vi "LVClass_WavefrontCorrector Get amplitude.vi"(0 "WavefrontCorrector in":refnum<class "WavefrontCorrector.lvclass">, 5 "Absolute Positions":T1, 11 "error in (no error)":errorcluster) -> (4 "WavefrontCorrector out":refnum<class "WavefrontCorrector.lvclass">, 6 "Absolute Positions OUT":T1, 8 "command_amplitude":sgl, 15 "error out":errorcluster)   [LabVIEW 2020, in "WavefrontCorrector.lvclass"]
doc: "Assert if requested absolute positions satisfy current preferences.\n\n--------------------------------------------------------------------------------\n\n<B>correctorIn </B> : WavefrontCorrector object.\n<B>correctorOut </B> : WavefrontCorrector object.\n<B>position </B> : Requested absolutes positions.\n<B>ErrorIn </B> : Error\n<B>ErrorOut </B> : Error\n\n--------------------------------------------------------------------------------"
uses:
  WavefrontCorrector.lvclass
  Wavefront Corrector Position.ctl
  WavefrontCorrector.lvclass/WavefrontCorrector.ctl
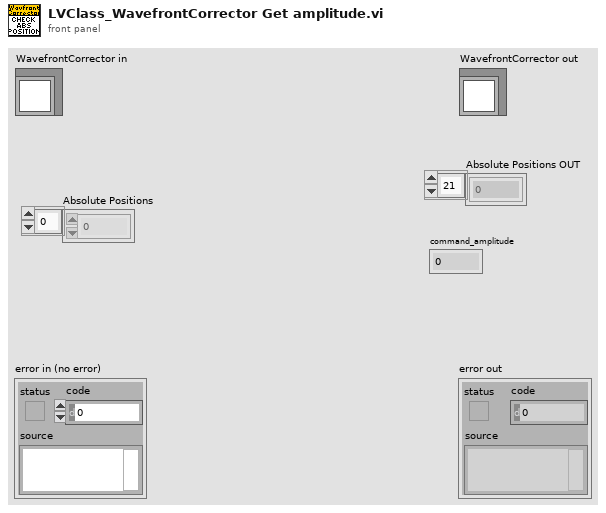
[diagram p1: front panel]
types:
  T1 = typedef "Wavefront Corrector Position.ctl" = sgl[]
  T2 = typedef "ClassID.ctl" = i64
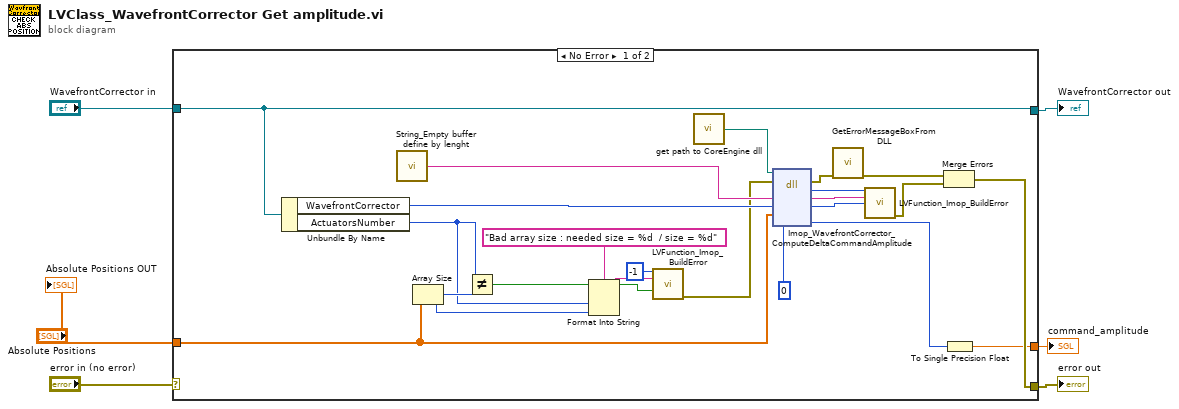
[diagram p0: block diagram]
diagram:
  n1 = case shown="No Error" "error in (no error)" {
    selector: "error in (no error)" -> [_ w30]
    tunnel: [w20 w30] -> w3
    tunnel: [w19 w29] -> w4
    tunnel: "WavefrontCorrector in" -> [w19 w29]
    tunnel: "Absolute Positions" -> [w11 _]
    tunnel: [w8 _] -> w1
    frame No Error {
      n2 = Unbundle By Name(w19) -> ("WavefrontCorrector"=w21:T2, "ActuatorsNumber"=w13:i32)
      n3 = call "String_Empty buffer define by lenght.vi"() -> ("Empty buffer"=w26:string)  [unwired: 1 in]
      n4 = Array Size(array=w11) -> (size(s)=w16:i32)
      n5 = Not Equal?(x=w13, y=w16) -> (x != y?=w15:bool)
      n6 = Format Into String(format string="Bad array size : needed size = %d  / size = %d" ("String to Prepend to source (\"\")"), w13, w16) -> (resulting string=w17:string)  [unwired: 2 in, 1 out]
      n7 = call "LVFunction_Imop_BuildError.vi"("code"=-1, "String to Prepend to source (\"\")"=w17, "Activate error? (true)"=w15) -> ("error out"=w12:errorcluster)  [unwired: 12 in]
      n8 = call "get path to CoreEngine dll.vi"() -> ("path to wavekit library"=w25:path)  [unwired: 14 in, 1 out]
      n9 = dll-call lib="D:/soft/HASO_v3/SVN_trunk/ImOpCoreEngine4_LV2011/DLLs/c_interface_vc100.dll" fn="Imop_WavefrontCorrector_ComputeDeltaCommandAmplitude"(path in=w25, error in=w12, "message"=w26, "WavefrontCorrection"=w21, "position"=w11, "command_amplitude"=0) -> (error out=w24:errorcluster, "return type"=w28:i32, "message"=w27:string, "WavefrontCorrection"=w7:i64, "command_amplitude"=w10:i32)  [unwired: 2 in, 1 out]
      n10 = call "GetErrorMessageBoxFromDLL.vi"("error IN"=w24) -> ("error OUT"=w23:errorcluster)  [unwired: 10 in]
      n11 = call "LVFunction_Imop_BuildError.vi"("code"=w28, "String to Prepend to source (\"\")"=w27, "Adresse"=w7) -> ("error out"=w22:errorcluster)  [unwired: 12 in]
      n12 = Merge Errors(w23, w22) -> (w20:errorcluster)
      n13 = To Single Precision Float(number=w10) -> (single precision float=w8:sgl)
    }
    frame Error {
    }
  }
  "error out" <- w3
  "WavefrontCorrector out" <- w4
  "command_amplitude" <- w1
  "Absolute Positions OUT" <- "Absolute Positions"
